vi "HPButterworthFilter.vi"(2 "order":u8=2, 3 "Cutoff Radius":dbl=0.5 min=0.0 max=1.0 format="%.2f", 4 "Image In":T1 {"Dialogs" format="%.0b"}) -> (0 "FFT Out":T1 {"Dialogs" format="%.0b"}, 1 "Image Out":T1 {"Dialogs" format="%.0b"})   [LabVIEW 2024]
doc: "This VI applies a Low Pass Butterworth filter in the frequency domain. The cutoff ratio is expressed as a percentage of the maximum radius. It only works on greyscale images."
uses:
  <userlib>/ImageProcessing/QTLIB_2595_LV86/QT_Image.ctl
panel:
  # "This VI applies a Low Pass Butterworth filter in the frequency domain.  The cutoff ratio is expressed as a percentage of the maximum radius. It only works on greyscale images."
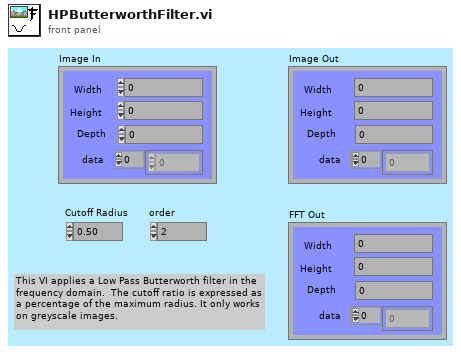
[diagram p1: front panel]
types:
  T1 = typedef "QT_Image.ctl" = cluster{"Width":i32, "Height":i32, "Depth":i32, "data":u8[], "Compressed data":u8[], "Color table":u32[], "Duration":i32, "Options":i32, "Timestamp":i32, "ID":i32, "Reserved":i32, "Dialogs":u32}
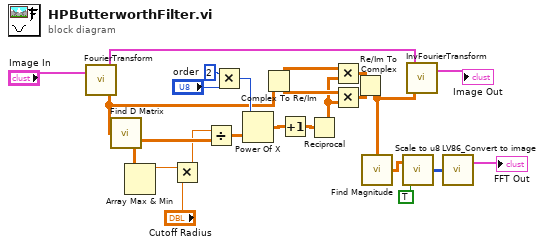
[diagram p0: block diagram]
diagram:
  n1 = call <userlib>:"FourierTransform.vi"("Image In"="Image In") -> ("Complex FT"=w5:cdb[][], "Image Out"=w24:T1)  [unwired: 1 in]
  n2 = call <userlib>:"Find D Matrix.vi"("Complex FT"=w5) -> ("Intensity Graph"=w11:dbl[][])
  n3 = Array Max & Min(array=w11) -> (max value=w10:dbl)  [unwired: 3 out]
  n4 = Multiply(x=w10, y="Cutoff Radius") -> (x*y=w9:dbl)
  n5 = Divide(x=w9, y=w11) -> (x/y=w19:dbl[][])
  n6 = Multiply(x=2, y="order") -> (x*y=w17:i32)
  n7 = Power Of X(1:w19, 2:w17) -> (0:w16:dbl[][])
  n8 = Complex To Re/Im(x + iy=w5) -> (x=w7:dbl[][], y=w6:dbl[][])
  n9 = Increment(x=w16) -> (x+1=w15:dbl[][])
  n10 = Reciprocal(x=w15) -> (1/x=w4:dbl[][])
  n11 = Multiply(x=w7, y=w4) -> (x*y=w3:dbl[][])
  n12 = Multiply(x=w6, y=w4) -> (x*y=w2:dbl[][])
  n13 = Re/Im To Complex(1:w2, 2:w3) -> (0:w1:cdb[][])
  n14 = call <userlib>:"Find Magnitude.vi"("FFT {X}"=w1) -> ("Magnitude"=w21:dbl[][])
  n15 = call <userlib>:"Scale to u8.vi"("Log scaling?"=TRUE, "Intensity Graph"=w21) -> ("X"=w22:u8[][])
  n16 = call <userlib>:"InvFourierTransform.vi"("Complex matrix"=w1, "Image In"=w24) -> ("Image Out"=→"Image Out":T1)  [unwired: 1 in]
  n17 = call <userlib>:"LV86_Convert to image.vi"("Intensity Graph"=w22) -> ("Image Out"=→"FFT Out":T1)  [unwired: 2 in]
